vi "Init.vi"(8 "error in (no error)":errorcluster, 9 "Config File Path":path=path "", 10 "Name":string, 11 "View In":refnum<class "View.lvclass">) -> (0 "error out":errorcluster, 3 "View Out":refnum<class "View.lvclass">)   [LabVIEW 2020, in "View.lvclass"]
doc: "Initializes the process and creates necessary references. Anything initialized here is released in the Clear.vi method."
uses:
  View.lvclass
  View.lvclass/View.ctl
  Process/Process.lvclass
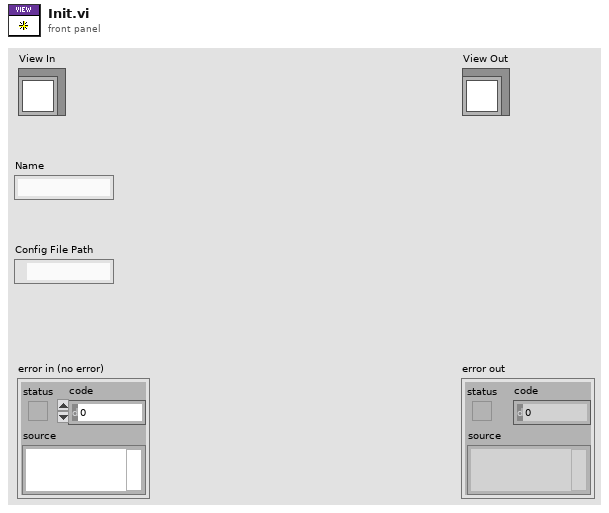
[diagram p1: front panel]
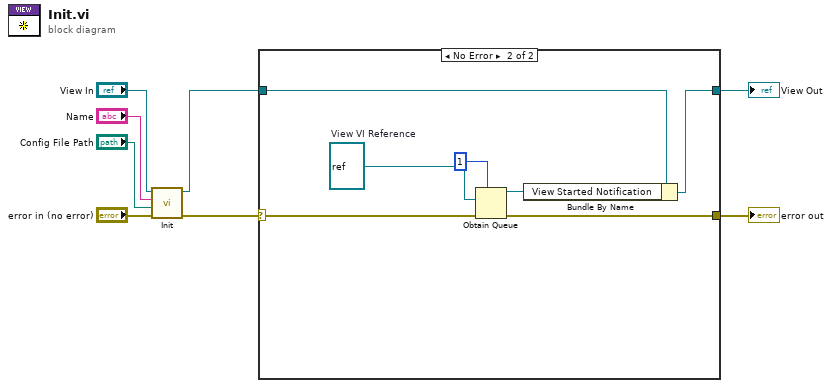
[diagram p0: block diagram]
diagram:
  n1 = call-parent "Init.vi"("error in (no error)"="error in (no error)", "Config File Path"="Config File Path", "Name"="Name", "Process In"="View In") -> ("error out"=w1:errorcluster, "Process Out"=w2:refnum<class "View.lvclass">)  [unwired: 6 in]
  n2 = case shown="No Error" w1 {
    selector: w1 -> [w9 w14]
    tunnel: [w10 w17] -> w4
    tunnel: [w9 w15] -> w3
    tunnel: w2 -> [w10 w13]
    frame Default {
    }
    frame No Error {
      w16 = refnum<vi> refnum  # View VI Reference
      n3 = Obtain Queue(max queue size (-1, unlimited)=1, element data type=w16, error in (no error)=w14) -> (queue out=w12:refnum<queue>, error out=w15:errorcluster)  [unwired: 2 in, 1 out]
      n4 = Bundle By Name(cluster=w13, "View Started Notification"=w12) -> (w17:refnum<class "View.lvclass">)
    }
  }
  "error out" <- w3
  "View Out" <- w4
